vi "new aggregate dialog.vi"(11 "Countries":string[](array[string])) -> ()   [LabVIEW 2019]
uses:
  <vilib>/Utility/sysdir.llb/System Directory Type.ctl
  <vilib>/Utility/config.llb/Write Key (String).vi
  <vilib>/Utility/config.llb/Read Key (String).vi
  <vilib>/Utility/config.llb/NI_LVConfig.lvlib
panel:
  in  "existing aggregates":string(combo)
  in  "Aggregate name":string
  in  "Cancel Button":bool
  in  "Save Button":bool
  in  "Remove Button":bool
  in  "Add Button":bool
  in  "New Agregate":i32(listbox)
  in  "Select Country":i32[](listbox)
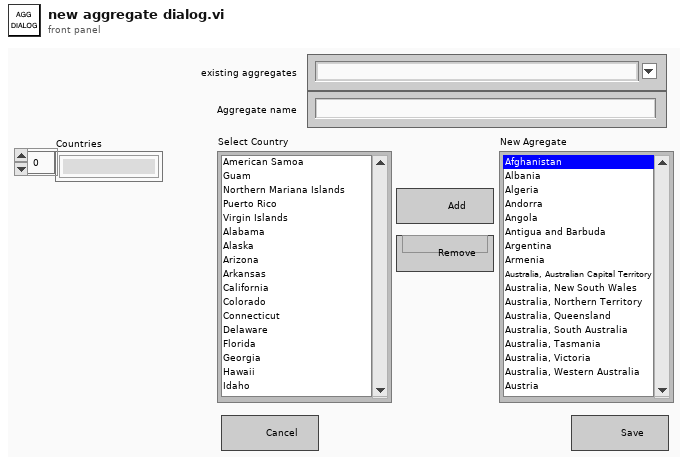
[diagram p1: front panel]
types:
  T1 = typedef "System Directory Type.ctl" = i32
  T2 = typedef "NI_LVConfig.lvlib/Config Data RefNum.ctl" = refnum<k1>
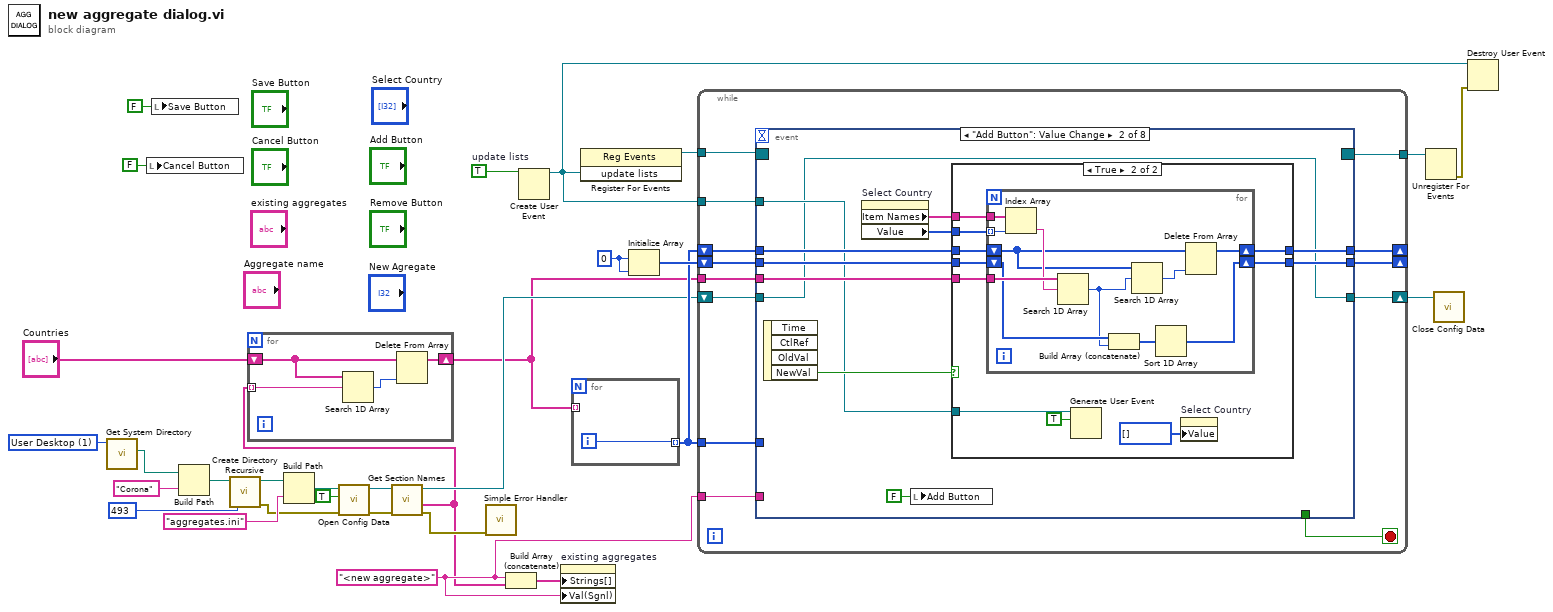
[diagram p0: block diagram]
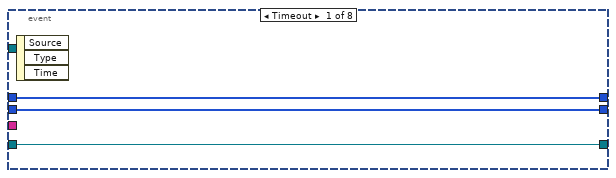
[diagram p2: hidden frame]
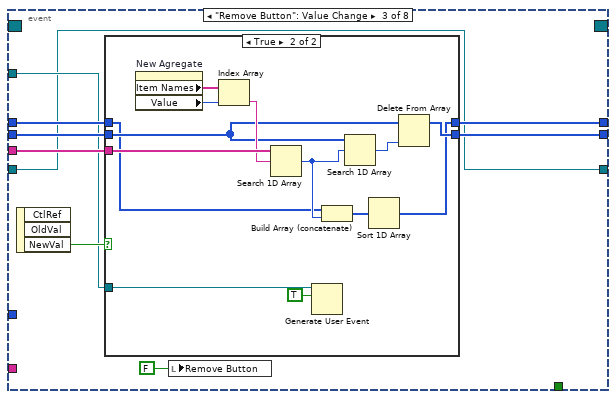
[diagram p4: hidden frame]
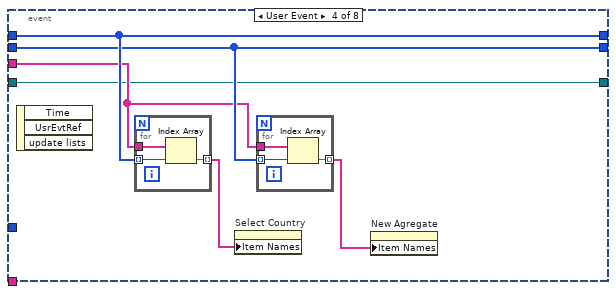
[diagram p6: hidden frame]
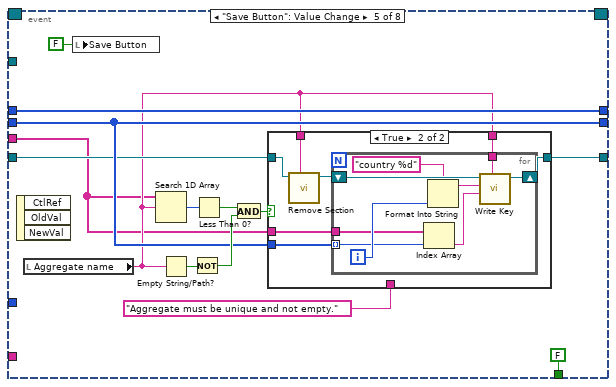
[diagram p7: hidden frame]
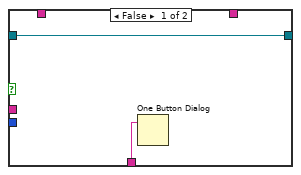
[diagram p8: hidden frame]
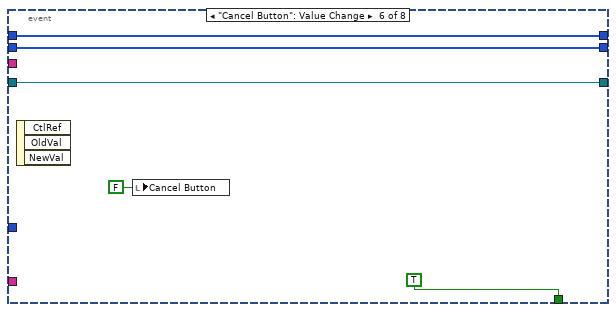
[diagram p9: hidden frame]
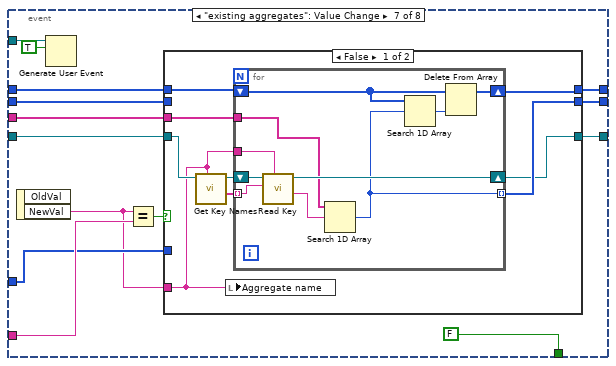
[diagram p10: hidden frame]
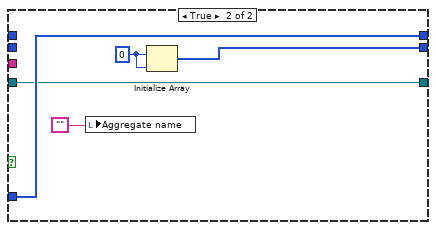
[diagram p11: hidden frame]
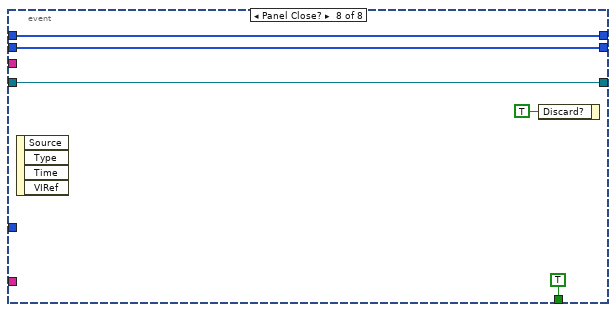
[diagram p12: hidden frame]
diagram:
  w6 = "<new aggregate>"
  w23 = T1 1 items=["User Home"=0, "User Desktop"=1, "User Documents"=2, "User Application Data"=3, "User Preferences"=4, "User Temporary"=5, "Public Documents"=6, "Public Application Data"=7, "Public Preferences"=8, "Public Cache"=13, "System Core Libraries"=9, "System Installed Libraries"=10, "Application Files"=11, "Boot Volume Root"=12] ("system directory type")
  w27 = TRUE  # update lists
  w30 = 0
  n1 = call <vilib>:"Get System Directory.vi"("system directory type"=w23) -> ("system directory"=w22:path)  [unwired: 10 in]
  n2 = local write "Cancel Button"(FALSE ("Cancel Button")) -> ()
  n3 = local write "Save Button"(FALSE ("Save Button")) -> ()
  n4 = Build Path(base path=w22, name or relative path="Corona") -> (appended path=w14:path)
  n5 = call <vilib>:"Create Directory Recursive.vi"("permissions"=i16 493, "directory"=w14) -> ("error out"=w12:errorcluster, "directory copy"=w13:path)  [unwired: 3 in, 1 out]
  n6 = Build Path(base path=w13, name or relative path="aggregates.ini") -> (appended path=w19:path)
  n7 = call <vilib>:"Open Config Data.vi"("error in (no error)"=w12, "create file if necessary (T)"=TRUE, "configuration file path"=w19) -> ("error out"=w16:errorcluster, "refnum"=w17:T2)  [unwired: 6 in, 1 out]
  n8 = call <vilib>:"Get Section Names.vi"("error in (no error)"=w16, "refnum"=w17) -> ("error out"=w15:errorcluster, "section names"=w4:string[], "refnum out"=w8:T2)  [unwired: 7 in]
  n9 = for {
    shift-right: [w34] -> w3
    shift-left: "Countries" -> [w32]
    tunnel: w4 -> [w33] mode=indexing
    n10 = Search 1D Array(1D array=w32, element=w33) -> (index of element=w31:i32)  [unwired: 1 in]
    n11 = Delete From Array(array=w32, index=w31) -> (array with subset deleted=w34:string[])  [unwired: 1 in, 1 out]
  }
  n12 = call <vilib>:"Simple Error Handler.vi"("error in (no error)"=w15) -> ()  [unwired: 4 in, 5 out]
  n13 = Build Array (concatenate)(w6, w4) -> (w10:string[])
  n14 = Create User Event(user event datatype=w27) -> (user event=w25:refnum<user-event>)  [unwired: 1 in, 1 out]
  n15 = property on="existing aggregates" class="CmbBox"("Strings[]"=w10, "Val(Sgnl)"=w6) -> ()  [unwired: 2 in, 2 out]
  n16 = for {
    tunnel: w3 -> [_] mode=indexing
    tunnel: [w35] -> w9 mode=indexing
    i -> [w35]
  }
  n17 = register-events(w25) -> (reference out=w28:refnum<event-registration>)  [unwired: 2 in, 1 out]
  n18 = Initialize Array(w30, w30) -> (w29:i32[])
  n19 = while {
    shift-right: [w46] -> _
    shift-left: w9 -> [w48]
    tunnel: w3 -> [w47]
    shift-right: [w44] -> _
    shift-left: w29 -> [w45]
    tunnel: w28 -> [w43]
    tunnel: w25 -> [w42]
    tunnel: [w41] -> w26
    tunnel: w6 -> [w39]
    tunnel: w9 -> [w38]
    shift-right: [w36] -> w7
    shift-left: w8 -> [w37]
    stop <- w40 stop-if-true
    n20 = event shown="[1] \"Add Button\": Value Change" {
      selector: w43 -> [_ _ _ _ _ _ _ _]
      dyn-events: [_ _ _ _ _ _ _ _] -> w41
      timeout: _ -> [_ _ _ _ _ _ _ _]
      tunnel: w48 -> [w51 w60 w92 w115 w135 w158 w170 w201]
      tunnel: w47 -> [_ w59 w91 w113 w123 _ w159 _]
      tunnel: [w51 w58 w90 w115 w135 w158 w169 w201] -> w46
      tunnel: w45 -> [w50 w57 w89 w114 w127 w157 w168 w200]
      tunnel: [w50 w56 w88 w114 w127 w157 w167 w200] -> w44
      tunnel: w42 -> [_ w55 w87 _ _ _ w164 _]
      tunnel: [_ _ _ _ FALSE TRUE FALSE TRUE] -> w40
      tunnel: w39 -> [_ _ _ _ _ _ w171 _]
      tunnel: w38 -> [_ _ _ _ _ _ w165 _]
      tunnel: w37 -> [w49 w54 w86 w110 w126 w155 w161 w199]
      tunnel: [w49 w54 w86 w110 w125 w155 w160 w199] -> w36
      event Timeout {
        n21 = event-data() -> ()  [unwired: 1 in, 3 out]
      }
      event "Add Button": Value Change {
        n22 = event-data() -> ("NewVal"=w62:bool)  [unwired: 1 in, 3 out]
        n23 = property on="Select Country" class="LstBox (strict)"() -> ("Item Names"=w53:string[], "Value"=w52:i32[])  [unwired: 2 in, 2 out]
        n24 = local write "Add Button"(FALSE ("Add Button")) -> ()
        n25 = case shown="True" w62 {
          tunnel: w60 -> [w64 w73]
          tunnel: w59 -> [_ w74]
          tunnel: [w64 w67] -> w58
          tunnel: w57 -> [w63 w72]
          tunnel: [w63 w68] -> w56
          tunnel: w55 -> [_ w71]
          tunnel: w53 -> [_ w69]
          tunnel: w52 -> [_ w66]
          frame False {
          }
          frame True {
            n26 = for {
              tunnel: w74 -> [w85]
              tunnel: w69 -> [w78]
              shift-right: [w76] -> w67
              shift-left: w73 -> [w82]
              shift-right: [w77] -> w68
              shift-left: w72 -> [w81]
              tunnel: w66 -> [w75] mode=indexing
              n27 = Index Array(array=w78, index=w75) -> (element=w84:string)
              n28 = Search 1D Array(1D array=w85, element=w84) -> (index of element=w80:i32)  [unwired: 1 in]
              n29 = Build Array (concatenate)(w81, w80) -> (w79:i32[])
              n30 = Search 1D Array(1D array=w82, element=w80) -> (index of element=w83:i32)  [unwired: 1 in]
              n31 = Sort 1D Array(array=w79) -> (sorted array=w77:i32[])
              n32 = Delete From Array(array=w82, index=w83) -> (array with subset deleted=w76:i32[])  [unwired: 1 in, 1 out]
            }
            n33 = Generate User Event(user event=w71, event data cluster=TRUE ("event data")) -> ()  [unwired: 2 in, 2 out]
            n34 = property on="Select Country" class="LstBox (strict)"("Value"=i32[] [] ("Select Country")) -> ()  [unwired: 2 in, 2 out]
          }
        }
      }
      event "Remove Button": Value Change {
        n35 = event-data() -> ("NewVal"=w94:bool)  [unwired: 1 in, 2 out]
        n36 = case shown="True" w94 {
          tunnel: w92 -> [w96 w100]
          tunnel: w91 -> [_ w107]
          tunnel: [w96 w99] -> w90
          tunnel: w89 -> [w95 w102]
          tunnel: [w95 w101] -> w88
          tunnel: w87 -> [_ w98]
          frame False {
          }
          frame True {
            n37 = property on="New Agregate" class="LstBox (strict)"() -> ("Item Names"=w108:string[], "Value"=w109:i32)  [unwired: 2 in, 2 out]
            n38 = Index Array(array=w108, index=w109) -> (element=w106:string)
            n39 = Search 1D Array(1D array=w107, element=w106) -> (index of element=w104:i32)  [unwired: 1 in]
            n40 = Generate User Event(user event=w98, event data cluster=TRUE ("event data")) -> ()  [unwired: 2 in, 2 out]
            n41 = Build Array (concatenate)(w100, w104) -> (w103:i32[])
            n42 = Search 1D Array(1D array=w102, element=w104) -> (index of element=w105:i32)  [unwired: 1 in]
            n43 = Sort 1D Array(array=w103) -> (sorted array=w99:i32[])
            n44 = Delete From Array(array=w102, index=w105) -> (array with subset deleted=w101:i32[])  [unwired: 1 in, 1 out]
          }
        }
        n45 = local write "Remove Button"(FALSE ("Add Button")) -> ()
      }
      event User Event {
        n46 = event-data() -> ()  [unwired: 1 in, 3 out]
        n47 = for {
          tunnel: w115 -> [w120] mode=indexing
          tunnel: w113 -> [w121]
          tunnel: [w119] -> w112 mode=indexing
          n48 = Index Array(array=w121, index=w120) -> (element=w119:string)
        }
        n49 = property on="Select Country" class="LstBox (strict)"("Item Names"=w112) -> ()  [unwired: 2 in, 2 out]
        n50 = for {
          tunnel: w114 -> [w117] mode=indexing
          tunnel: w113 -> [w118]
          tunnel: [w116] -> w111 mode=indexing
          n51 = Index Array(array=w118, index=w117) -> (element=w116:string)
        }
        n52 = property on="New Agregate" class="LstBox (strict)"("Item Names"=w111) -> ()  [unwired: 2 in, 2 out]
      }
      event "Save Button": Value Change {
        n53 = event-data() -> ()  [unwired: 1 in, 3 out]
        n54 = local read "Aggregate name"() -> (w124:string)
        n55 = local write "Save Button"(FALSE ("Save Button")) -> ()
        n56 = Search 1D Array(1D array=w123, element=w124) -> (index of element=w134:i32)  [unwired: 1 in]
        n57 = Empty String/Path?(string/path=w124) -> (empty?=w133:bool)
        n58 = Not(x=w133) -> (.not. x?=w131:bool)
        n59 = Less Than 0?(x=w134) -> (x < 0?=w132:bool)
        n60 = And(x=w132, y=w131) -> (x .and. y?=w130:bool)
        n61 = case shown="True" w130 {
          tunnel: "Aggregate must be unique and not empty." -> [w137 _]
          tunnel: w127 -> [_ w144]
          tunnel: w124 -> [_ w143]
          tunnel: w126 -> [w136 w141]
          tunnel: [w136 w142] -> w125
          tunnel: w124 -> [_ w139]
          tunnel: w123 -> [_ w138]
          frame False {
            n62 = One Button Dialog(message=w137) -> ()  [unwired: 1 in, 1 out]
          }
          frame True {
            n63 = call <vilib>:"Remove Section.vi"("section"=w139, "refnum"=w141) -> ("refnum out"=w140:T2)  [unwired: 7 in, 2 out]
            n64 = for {
              tunnel: w143 -> [w152]
              tunnel: w144 -> [w148] mode=indexing
              shift-right: [w149] -> w142
              shift-left: w140 -> [w153]
              tunnel: w138 -> [w146]
              i -> [w150]
              n65 = Index Array(array=w146, index=w148) -> (element=w147:string)
              n66 = Format Into String(format string="country %d" ("key"), w150) -> (resulting string=w151:string)  [unwired: 2 in, 1 out]
              n67 = call-poly <vilib>:"Write Key.vi"("section"=w152, "value"=w147, "key"=w151, "refnum"=w153) -> ("refnum out"=w149:T2)  [unwired: 5 in, 2 out]
            }
          }
        }
      }
      event "Cancel Button": Value Change {
        n68 = event-data() -> ()  [unwired: 1 in, 3 out]
        n69 = local write "Cancel Button"(FALSE ("Cancel Button")) -> ()
      }
      event "existing aggregates": Value Change {
        n70 = event-data() -> ("NewVal"=w162:string)  [unwired: 1 in, 1 out]
        n71 = Generate User Event(user event=w164, event data cluster=TRUE ("event data")) -> ()  [unwired: 2 in, 2 out]
        n72 = Equal?(x=w162, y=w171) -> (x = y?=w166:bool)
        n73 = case shown="False" w166 {
          tunnel: w170 -> [w175 _]
          tunnel: [w174 w194] -> w169
          tunnel: w168 -> [_ _]
          tunnel: [w179 w196] -> w167
          tunnel: w165 -> [_ w194]
          tunnel: w162 -> [w176 _]
          tunnel: w161 -> [w178 w192]
          tunnel: [w177 w192] -> w160
          tunnel: w159 -> [w173 _]
          frame False {
            n74 = call <vilib>:"Get Key Names.vi"("section"=w176, "refnum"=w178) -> ("key names"=w181:string[], "refnum out"=w180:T2)  [unwired: 6 in, 2 out]
            n75 = local write "Aggregate name"(w176) -> ()
            n76 = for {
              tunnel: w181 -> [w189] mode=indexing
              shift-right: [w190] -> w177
              shift-left: w180 -> [w191]
              tunnel: [w182] -> w179 mode=indexing
              tunnel: w176 -> [w188]
              shift-right: [w186] -> w174
              shift-left: w175 -> [w185]
              tunnel: w173 -> [w183]
              n77 = call-poly <vilib>:"Read Key.vi"("section"=w188, "key"=w189, "refnum"=w191) -> ("value"=w184:string, "refnum out"=w190:T2)  [unwired: 5 in, 2 out]
              n78 = Search 1D Array(1D array=w183, element=w184) -> (index of element=w182:i32)  [unwired: 1 in]
              n79 = Search 1D Array(1D array=w185, element=w182) -> (index of element=w187:i32)  [unwired: 1 in]
              n80 = Delete From Array(array=w185, index=w187) -> (array with subset deleted=w186:i32[])  [unwired: 1 in, 1 out]
            }
          }
          frame True {
            w195 = 0
            n81 = local write "Aggregate name"("") -> ()
            n82 = Initialize Array(w195, w195) -> (w196:i32[])
          }
        }
      }
      event Panel Close? {
        n83 = event-data() -> ()  [unwired: 1 in, 4 out]
        n84 = event-data("Discard?"=TRUE) -> ()  [unwired: 1 in, 1 out]
      }
    }
  }
  n85 = Unregister For Events(event registration refnum=w26) -> (error out=w24:errorcluster)  [unwired: 1 in]
  n86 = call <vilib>:"Close Config Data.vi"("refnum"=w7) -> ()  [unwired: 9 in, 2 out]
  n87 = Destroy User Event(user event=w25, error in=w24) -> ()  [unwired: 1 out]
